vi "rnd(span).vi"(10 "min":dbl, 11 "max":dbl) -> (2 "mapped":dbl, 5 "span":dbl)   [LabVIEW 2018, in "LV2Julia_core.lvlib"]
uses:
  LV2Julia_core.lvlib
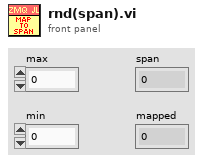
[diagram p1: front panel]
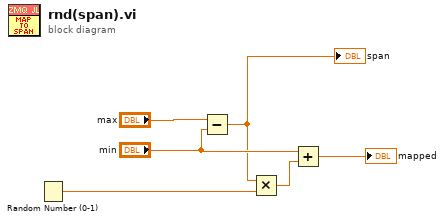
[diagram p0: block diagram]
diagram:
  n1 = Random Number (0-1)() -> (number: 0 to 1=w1:dbl)
  n2 = Subtract(x="max", y="min") -> (x-y=w3:dbl)
  "span" <- w3
  n3 = Multiply(x=w3, y=w1) -> (x*y=w4:dbl)
  n4 = Add(x="min", y=w4) -> (x+y=→"mapped":dbl)
